vi "sub_strain-cal2.vi"(11 "strain wfs":waveform(dbl)[](array[waveform])) -> (1 "force":dbl, 3 "force wf":waveform(dbl))   [LabVIEW 2016]
uses:
  <vilib>/Analysis/baseanly.llb/Mean (DBL).vi
  <vilib>/Analysis/NI_AALBase.lvlib
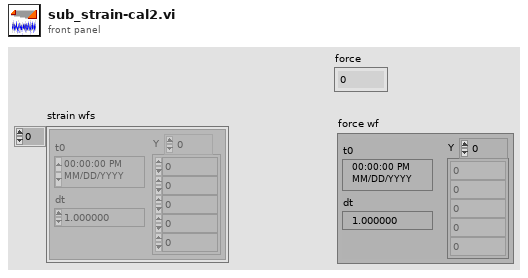
[diagram p1: front panel]
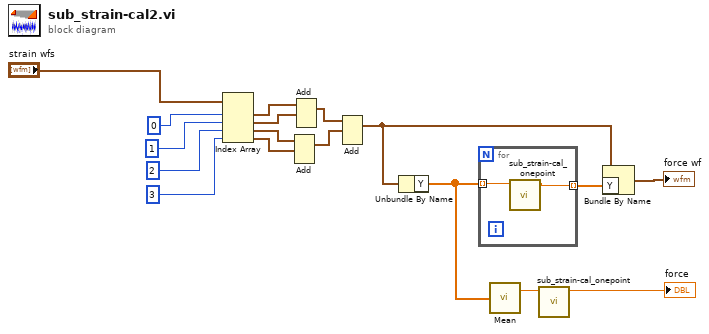
[diagram p0: block diagram]
diagram:
  n1 = Index Array(array="strain wfs", index #1=0 ("인덱스"), index #2=1 ("인덱스"), index #3=2 ("인덱스"), index #4=3 ("인덱스")) -> (element #1=w7:waveform(dbl), element #2=w6:waveform(dbl), element #3=w5:waveform(dbl), element #4=w4:waveform(dbl))
  n2 = Add(1:w4, 2:w5) -> (0:w2:waveform(dbl))  [unwired: 1 in, 1 out]
  n3 = Add(1:w6, 2:w7) -> (0:w3:waveform(dbl))  [unwired: 1 in, 1 out]
  n4 = Add(1:w2, 2:w3) -> (0:w1:waveform(dbl))  [unwired: 1 in, 1 out]
  n5 = Unbundle By Name(w1) -> ("Y"=w13:dbl[])
  n6 = for {
    tunnel: w13 -> [w19] mode=indexing
    tunnel: [w18] -> w16 mode=indexing
    n7 = call "sub_strain-cal_onepoint.vi"("strain"=w19) -> ("g force"=w18:dbl)  [unwired: 10 in]
  }
  n8 = call-poly <vilib>:"Mean.vi"("X"=w13) -> ("mean"=w14:dbl)  [unwired: 1 out]
  n9 = call "sub_strain-cal_onepoint.vi"("strain"=w14) -> ("g force"=→"force":dbl)  [unwired: 10 in]
  n10 = Bundle By Name(cluster=w1, "Y"=w16) -> (→"force wf":waveform(dbl))
